vi "Tank Drive.vi"() -> ()   [LabVIEW 2025]
doc: "Tank Drive Example\n\nThis example shows how to implement tank drive and uses two joysticks for input.\n\nThis example expects a USB cable connected from your development PC to the Type B USB Jack (next to the power input) on the roboRIO.\n\nThis example requires the Driver Station to be running with Teleoperated Enabled."
uses:
  <vilib>/Rock Robotics/SystemInterfaces/DIO/FPGA_DIOPWMChannel.ctl
  <vilib>/Rock Robotics/WPI/Joystick/WPI_JoystickDeviceEnum.ctl
  <vilib>/Rock Robotics/WPI/RobotDrive/WPI_RobotDriveOpen2MotorWithTalon.vi
panel:
  in  "RightStick":T1=enum."USB 1"
  in  "LeftStick":T1
  in  "Left Motor (PWM channel)":T2
  in  "Right Motor (PWM channel)":T2=enum."PWM 1"
  in  "stop":bool
  # "Set these inputs before running."
  # "This example requires the Driver Station to be running with Teleoperated Enabled."
  # "PWM cables"
  # "This shows wiring for Talon speed controllers.  The wiring is similar for other motor controllers.  If you change the controller type, you must also select the appropriate instance of the Motor Open VI on the diagram."
  # "Power\nTerminals"
  # "Motor\nTerminals"
  # "+"
  # "+"
  # "M"
  # "B"
  # "Power\nTerminals"
  # "Motor\nTerminals"
  # "+"
  # "+"
  # "M"
  # "B"
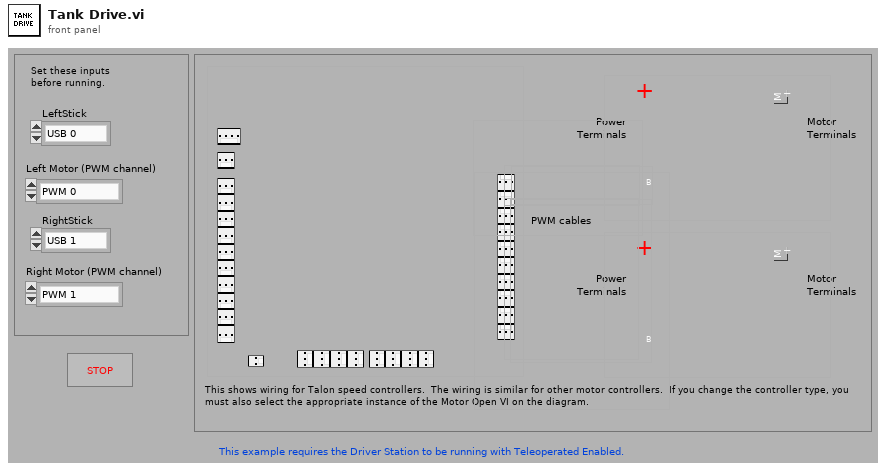
[diagram p1: front panel]
types:
  T1 = typedef "WPI_JoystickDeviceEnum.ctl" = enum16{"USB 0", "USB 1", "USB 2", "USB 3", "USB 4", "USB 5"}
  T2 = typedef "FPGA_DIOPWMChannel.ctl" = enum8{"PWM 0", "PWM 1", "PWM 2", "PWM 3", "PWM 4", "PWM 5", "PWM 6", "PWM 7", "PWM 8", "PWM 9", "PWM MXP 0", "PWM MXP 1", "PWM MXP 2", "PWM MXP 3", "PWM MXP 4", "PWM MXP 5", "PWM MXP 6", "PWM MXP 7", "PWM MXP 8", "PWM MXP 9", "Invalid"}
  T3 = typedef "WPI_JoystickDevRef.ctl" = cluster{"Device":T1}
  T4 = typedef "WPI_RobotDriveDevRef.ctl" = cluster{"DevStatus":errorcluster, "Motors[]":T5[], "Square Inputs":bool, "Max Output":dbl}
  T5 = typedef "WPI_MotorControlDeviceRef.ctl" = cluster{"DeviceStatus":errorcluster, "Type":T6, "PWM":cluster{"PWM Channel":T2, "DeadBand":T7}, "CAN":cluster{"Device Number":u8, "SetOutput VI Ref":variant, "GetOutput VI Ref":variant, "Enable VI Ref":variant, "Disable VI Ref":variant, "Data":variant}, "Invert":bool, "DIO PWM":cluster{"PWM \"Enable\" Channel":T2, "DIOChannel":T8, "PWM Rate":dbl}}
  T6 = typedef "WPI_MotorControlType.ctl" = enum16{"PWM", "CAN", "DIO PWM"}
  T7 = typedef "WPI_PWMDeadband.ctl" = cluster{"Name":string, "maxPositivePwm":i32, "minPositivePwm":i32, "centerPwm":i32, "maxNegativePwm":i32, "minNegativePwm":i32, "angularRange":u16}
  T8 = typedef "FPGA_DIOChannel.ctl" = enum8{"DIO 0", "DIO 1", "DIO 2", "DIO 3", "DIO 4", "DIO 5", "DIO 6", "DIO 7", "DIO 8", "DIO 9", "DIO MXP 0", "DIO MXP 1", "DIO MXP 2", "DIO MXP 3", "DIO MXP 4", "DIO MXP 5", "DIO MXP 6", "DIO MXP 7", "DIO MXP 8", "DIO MXP 9", "DIO MXP 10", "DIO MXP 11", "DIO MXP 12", "DIO MXP 13", "DIO MXP 14", "DIO MXP 15", "SPI Port CS1", "SPI Port CS2", "SPI Port CS3", "SPI Port MISO", "SPI Port MOSI", "Invalid"}
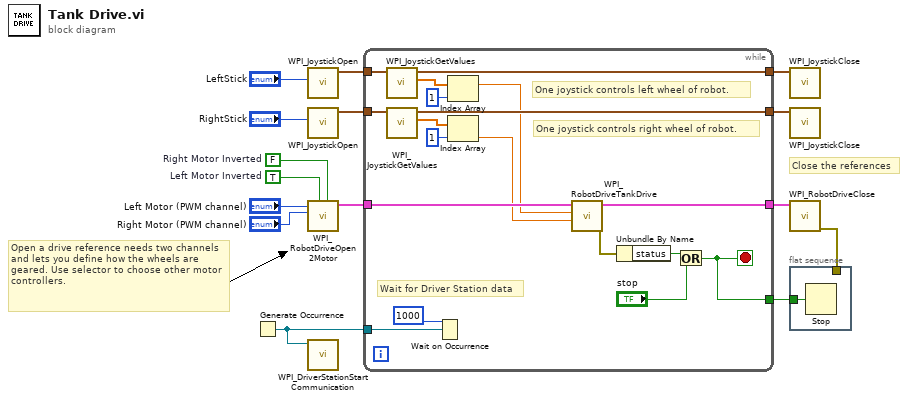
[diagram p0: block diagram]
diagram:
  w9 = FALSE  # Right Motor Inverted
  w10 = TRUE  # Left Motor Inverted
  # "Close the references"
  # "Open a drive reference needs two channels and lets you define how the wheels are geared. Use selector to choose other motor controllers."
  n1 = Generate Occurrence() -> (w11:refnum<k4>)
  n2 = call <vilib>:"WPI_JoystickOpen.vi"("JoystickDevice"="LeftStick") -> ("JoystickDevRef"=w5:T3)  [unwired: 10 out]
  n3 = call <vilib>:"WPI_JoystickOpen.vi"("JoystickDevice"="RightStick") -> ("JoystickDevRef"=w6:T3)  [unwired: 10 out]
  n4 = call-poly <vilib>:"WPI_RobotDriveOpen2Motor.vi"("Right Motor Inverted"=w9, "Left Motor Inverted"=w10, "Right Motor"="Right Motor (PWM channel)", "Left Motor"="Left Motor (PWM channel)") -> ("RobotDriveDevRef"=w13:T4)  [unwired: 1 in, 6 out]
  n5 = call <vilib>:"WPI_DriverStationStart Communication.vi"("occurrence"=w11) -> ()  [unwired: 2 in, 9 out]
  n6 = while {
    tunnel: w13 -> [w29]
    tunnel: [w19] -> w12
    tunnel: w11 -> [w33]
    tunnel: [w16] -> w2
    tunnel: w6 -> [w31]
    tunnel: w5 -> [w30]
    tunnel: [w27] -> w4
    tunnel: [w26] -> w3
    stop <- w16 stop-if-true
    # "Wait for Driver Station data"
    # "One joystick controls right wheel of robot."
    # "One joystick controls left wheel of robot."
    n7 = call <vilib>:"WPI_JoystickGetValues.vi"("JoystickDevRef"=w30) -> ("Axes"=w28:dbl[], "JoystickDevRef"=w27:T3)  [unwired: 6 in, 3 out]
    n8 = call <vilib>:"WPI_JoystickGetValues.vi"("JoystickDevRef"=w31) -> ("Axes"=w22:dbl[], "JoystickDevRef"=w26:T3)  [unwired: 6 in, 3 out]
    n9 = Wait on Occurrence(2:w33, 3:1000 ("ms timeout (-1)")) -> ()  [unwired: 2 out]
    n10 = Index Array(array=w28, index=1) -> (element=w25:dbl)
    n11 = Index Array(array=w22, index=1) -> (element=w21:dbl)
    n12 = call <vilib>:"WPI_RobotDriveTankDrive.vi"("Right axis value"=w21, "Left axis value"=w25, "RobotDriveDevRef"=w29) -> ("error out"=w18:errorcluster, "RobotDriveDevRef"=w19:T4)  [unwired: 1 in, 6 out]
    n13 = Unbundle By Name(w18) -> ("status"=w20:bool)
    n14 = Or(x=w20, y="stop") -> (x .or. y?=w16:bool)
  }
  n15 = call <vilib>:"WPI_JoystickClose.vi"("JoystickDevRef"=w4) -> ()  [unwired: 11 out]
  n16 = call <vilib>:"WPI_JoystickClose.vi"("JoystickDevRef"=w3) -> ()  [unwired: 11 out]
  n17 = call <vilib>:"WPI_RobotDriveClose.vi"("RobotDriveDevRef"=w12) -> ("error out"=w1:errorcluster)  [unwired: 1 in, 9 out]
  n18 = flat-sequence {
    tunnel: w2 -> [w34]
    tunnel: w1 -> [_]
    frame #0 {
      n19 = Stop(stop? (T)=w34) -> ()
    }
  }
